vi "Type Name Dialog.vi"(0 "Type Name:":string) -> (4 "Type Name Out":string, 8 "Cancelled?":bool)   [LabVIEW 2019]
panel:
  in  "Cancel":bool
  in  "OK":bool
  # "Enter a Type Name"
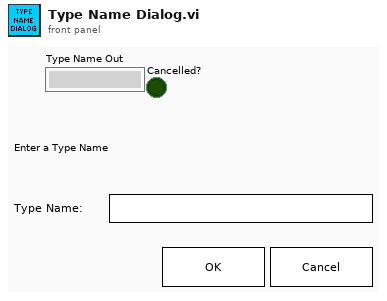
[diagram p1: front panel]
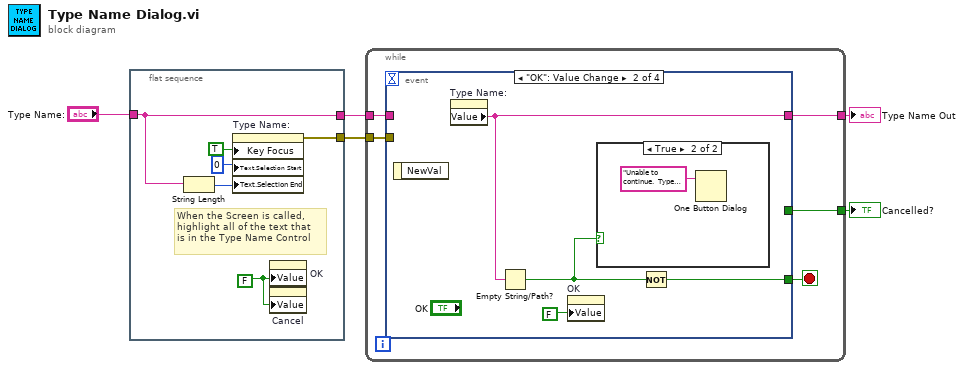
[diagram p0: block diagram]
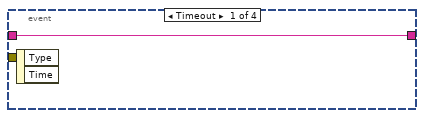
[diagram p2: hidden frame]
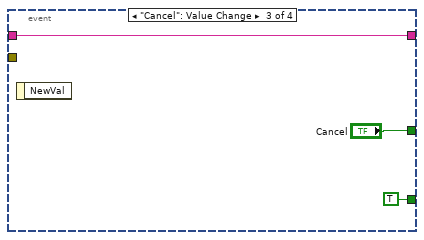
[diagram p4: hidden frame]
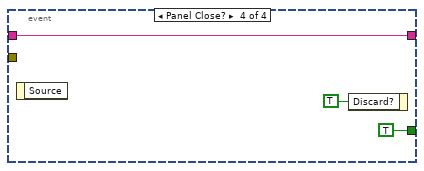
[diagram p5: hidden frame]
diagram:
  n1 = flat-sequence {
    tunnel: [w8] -> w3
    tunnel: [w7] -> w2
    tunnel: "Type Name:" -> [w7]
    frame #0 {
      w6 = FALSE ("Key Focus")
      # "When the Screen is called,\nhighlight all of the text that\nis in the Type Name Control"
      n2 = String Length(string=w7) -> (length=w10:i32)
      n3 = property on="Type Name:" class="Str"("Key Focus"=TRUE, "Text.Selection Start"=u32 0 ("Text.Selection:Start"), "Text.Selection End"=w10) -> (error out=w8:errorcluster)  [unwired: 2 in, 1 out]
      n4 = property on="OK" class="Bool (strict)"("Value"=w6) -> ()  [unwired: 2 in, 2 out]
      n5 = property on="Cancel" class="Bool (strict)"("Value"=w6) -> ()  [unwired: 2 in, 2 out]
    }
  }
  n6 = while {
    tunnel: [w16] -> w5
    tunnel: [w15] -> w4
    tunnel: w3 -> [w14]
    tunnel: w2 -> [w13]
    stop <- w12 stop-if-true
    n7 = event shown="[1] \"OK\": Value Change" {
      selector: _ -> [_ _ _ _]
      dyn-events: _ -> [_ _ _ _]
      timeout: _ -> [_ _ _ _]
      tunnel: w13 -> [w17 _ w24 w27]
      tunnel: [_ _ "Cancel" TRUE ("Cancel")] -> w16
      tunnel: [w17 w21 w24 w27] -> w15
      tunnel: w14 -> [_ _ _ _]
      tunnel: [_ w19 TRUE _] -> w12
      event Timeout {
        n8 = event-data() -> ()  [unwired: 1 in, 2 out]
      }
      event "OK": Value Change {
        n9 = event-data() -> ()  [unwired: 1 in, 1 out]
        n10 = property on="Type Name:" class="Str"() -> ("Value"=w21:string)  [unwired: 2 in, 2 out]
        n11 = Empty String/Path?(string/path=w21) -> (empty?=w20:bool)
        n12 = property on="OK" class="Bool (strict)"("Value"=FALSE ("Key Focus")) -> ()  [unwired: 2 in, 2 out]
        n13 = case shown="True" w20 {
          frame False {
          }
          frame True {
            n14 = One Button Dialog(message="Unable to continue.  Type Name must not be empty.") -> ()  [unwired: 1 in, 1 out]
          }
        }
        n15 = Not(x=w20) -> (.not. x?=w19:bool)
      }
      event "Cancel": Value Change {
        n16 = event-data() -> ()  [unwired: 1 in, 1 out]
      }
      event Panel Close? {
        n17 = event-data() -> ()  [unwired: 1 in, 1 out]
        n18 = event-data("Discard?"=TRUE) -> ()  [unwired: 1 in, 1 out]
      }
    }
  }
  "Cancelled?" <- w5
  "Type Name Out" <- w4
